vi "Get All Values from Config.vi"(8 "error in (no error)":errorcluster, 10 "Config name":string, 11 "Config in":refnum<class "Config.lvclass">) -> (0 "error out":errorcluster, 2 "All Parameters":string[][](array[string]), 3 "Config out":refnum<class "Config.lvclass">)   [LabVIEW 2026, in "TALOS.lvlib" / "Classes.lvlib" / "Config.lvclass"]
doc: "Returns a list of parameters with values for the specified configuration. If no configuration is provided, it use the Current Config."
uses:
  Config.lvclass
  Config.lvclass/Config.ctl
  Ancestor/Ancestor/Ancestor.lvclass/Ancestor.ctl
  FGV/Error Memory/Get Error Description.vi
  Support VIs/Get PC name.vi
  Ancestor/Ancestor/Read ID.vi
  Support VIs/Get Class Name.vi
  <vilib>/Utility/error.llb/Clear Errors.vi
  FGV/Error Memory/Error Memory Core.vi
  <vilib>/AdvancedString/Delimited String to 1D String Array.vi
  <vilib>/AdvancedString/Delimited String to 1D String Array (string).vi
  Support VIs/Circus Root Path.vi
  FGV/Error Memory/Error Crt Lvl checker.vi
  FGV/Error Memory/Error Memory Core.vi/40c8088d-b597-4017-91af-faa98e00292e.vi
  FGV/Error Memory/Error Memory Core.vi/d4a3ab98-063c-4e44-b43d-fbdcfe6c2be2.vi
  Support VIs/Global Memory.vi
  <vilib>/Utility/LVClass/Get LV Class Name.vi
  Support VIs/Is in Packed Library.vi
  Support VIs/TALOS Root path.vi
  Support VIs/Read CSV worksheet.vi
  Support VIs/Global Constants.vi
  <vilib>/Utility/error.llb/General Error Handler.vi
  Ancestor/Ancestor/Ancestor.lvclass
  <vilib>/Comparison/Equal/Equal Functor/Equal Functor.lvclass
  TALOS.lvlib
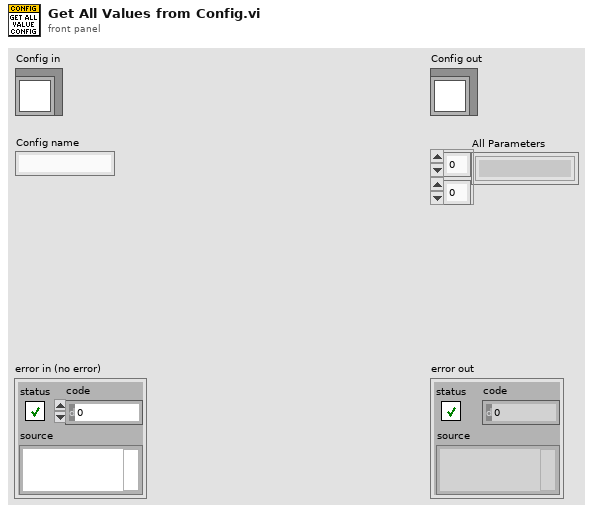
[diagram p1: front panel]
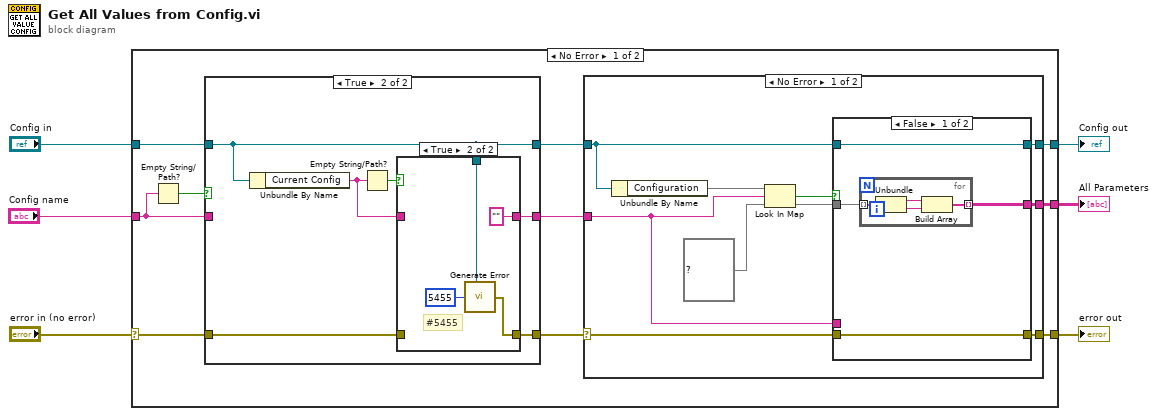
[diagram p0: block diagram]
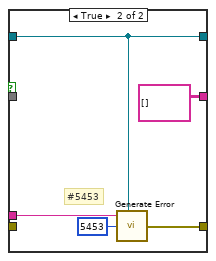
[diagram p2: hidden frame]
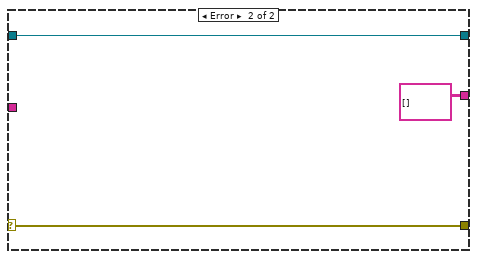
[diagram p3: hidden frame]
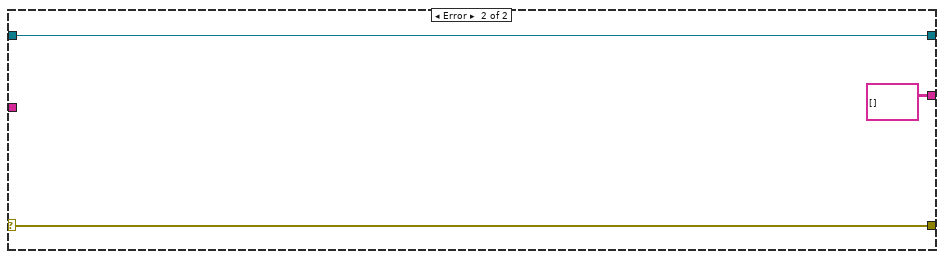
[diagram p6: hidden frame]
diagram:
  n1 = case shown="No Error" "error in (no error)" {
    selector: "error in (no error)" -> [w13 w60]
    tunnel: [w16 w60] -> w5
    tunnel: [w15 w59] -> w3
    tunnel: "Config in" -> [w14 w59]
    tunnel: "Config name" -> [w11 _]
    tunnel: [w7 string[][] [] ("Parameters")] -> w1
    frame No Error {
      n2 = Empty String/Path?(string/path=w11) -> (empty?=w12:bool)
      n3 = case shown="True" w12 {
        tunnel: w14 -> [w45 w46]
        tunnel: w13 -> [w43 w48]
        tunnel: w11 -> [w44 _]
        tunnel: [w45 w46] -> w10
        tunnel: [w44 w49] -> w9
        tunnel: [w43 w47] -> w8
        frame False {
        }
        frame True {
          n4 = Unbundle By Name(w46) -> ("Current Config"=w50:string)
          n5 = Empty String/Path?(string/path=w50) -> (empty?=w51:bool)
          n6 = case shown="True" w51 {
            tunnel: w50 -> [w53 _]
            tunnel: [w53 "" ("Current Config")] -> w49
            tunnel: w48 -> [w52 _]
            tunnel: [w52 w57] -> w47
            tunnel: w46 -> [_ w55]
            frame False {
            }
            frame True {
              # "#5455"
              n7 = call "Generate Error.vi"("Class"=w55, "Error Code"=5455) -> ("error out"=w57:errorcluster)  [unwired: 5 in]
            }
          }
        }
      }
      n8 = case shown="No Error" w8 {
        selector: w8 -> [w20 w41]
        tunnel: [w24 w41] -> w16
        tunnel: [w23 w42] -> w15
        tunnel: w10 -> [w22 w42]
        tunnel: w9 -> [w21 _]
        tunnel: [w18 string[][] [] ("Parameters")] -> w7
        frame No Error {
          n9 = Unbundle By Name(w22) -> ("Configuration"=w26:map{string, map{string, string}})
          n10 = Look In Map(map=w26, key=w21, default value=map{string, string} {}) -> (key not found?=w25:bool, value=w19:map{string, string})
          n11 = case shown="False" w25 {
            tunnel: w21 -> [_ w39]
            tunnel: [w30 w37] -> w24
            tunnel: w22 -> [w29 w35]
            tunnel: [w29 w35] -> w23
            tunnel: w20 -> [w30 _]
            tunnel: w19 -> [w28 _]
            tunnel: [w27 string[][] [] ("Parameters")] -> w18
            frame False {
              n12 = for {
                tunnel: w28 -> [w34] mode=indexing
                tunnel: [w31] -> w27 mode=indexing
                n13 = Unbundle(w34) -> ("Key"=w33:string, "Value"=w32:string)
                n14 = Build Array(w33, w32) -> (w31:string[])
              }
            }
            frame True {
              # "#5453"
              n15 = call "Generate Error.vi"("Optional String"=w39, "Class"=w35, "Error Code"=5453) -> ("error out"=w37:errorcluster)  [unwired: 4 in]
            }
          }
        }
        frame Error {
        }
      }
    }
    frame Error {
    }
  }
  "error out" <- w5
  "Config out" <- w3
  "All Parameters" <- w1
